vi "ShapeokoV3.vi"() -> ()   [LabVIEW 2024]
uses:
  <vilib>/Instr/_visa.llb/VISA Configure Serial Port (Instr).vi
  Subs/ShapekoGlobal.vi
panel:
  out "position":cluster{"X (inch)":dbl, "Y (inch)":dbl} {"X (inch)" format="%#.2g"; "Y (inch)" format="%#.2g"}
  out "position":cluster{"X (mm)":dbl, "Y (mm)":dbl}
  out "unlocked":bool
  in  "desired":cluster{"X":dbl, "Y":dbl, "Z":dbl}
  in  "Controls":T1
  in  "Jog":T2={"X-"=FALSE, "X+"=FALSE, "Y-"=FALSE, "Y+"=FALSE, "Z_"=FALSE, "Z+"=FALSE, "Dist"=1000, "Feed"=500} {"Feed" items=["100 mm/min"=100, "200 mm/min"=200, "300 mm/min"=300, "400 mm/min"=400, "500 mm/min"=500]; "Dist" items=["0.1 mm"=1, "1 mm"=10, "10 mm"=100, "100 mm"=1000]}
  in  "SubCut":cluster{dbl, dbl}(slide)={1.0, 0.0} scale=0.0..1.0
  out "(inch)":T3 {"Z Max" format="%#.3f"; "Z Min" format="%#.3f"; "Y Max" format="%#.3f"; "Y Min" format="%#.3f"; "X Max" format="%#.3f"; "X Min" format="%#.3f"}
  in  "Setup":T4={"Scaling (pixels/mm)"=1.0, "Tool Diameter (inch)"=0.25, "Origin location"={"x (mm)"=10, "y (mm)"=300}, "Wood dim"={"width (inch)"=10.0, "height (inch)"=12.0}}
  out "Tool Loc":picture
  in  "Path":path
  in  "Run":bool
  out "Cut":picture
  out "Bounds (mm)":T3 {"Z Max" format="%#.1f"; "Z Min" format="%#.1f"; "Y Max" format="%#.1f"; "Y Min" format="%#.1f"; "X Max" format="%#.1f"; "X Min" format="%#.1f"}
  out "Position":T5
  in  "stop":bool
  in  "VISA":refnum<visa-resource-name>="ASRL3::INSTR"
  in  "Cmds":i32(listbox)=-1
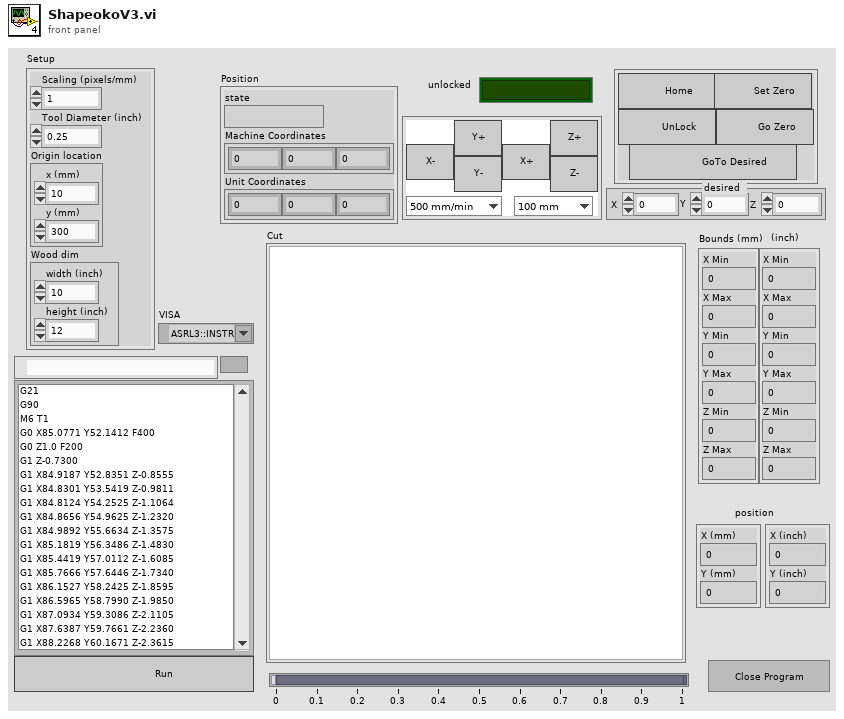
[diagram p1: front panel]
types:
  T1 = cluster{"Home Button":bool, "Set zero":bool, "Lock Button":bool, "Goto Zero":bool, "Goto Desired":bool}
  T2 = cluster{"X-":bool, "X+":bool, "Y-":bool, "Y+":bool, "Z_":bool, "Z+":bool, "Dist":u16, "Feed":u16}
  T3 = cluster{"X Min":dbl, "X Max":dbl, "Y Min":dbl, "Y Max":dbl, "Z Min":dbl, "Z Max":dbl}
  T4 = cluster{"Scaling (pixels/mm)":dbl, "Tool Diameter (inch)":dbl, "Origin location":cluster{"x (mm)":i16, "y (mm)":i16}, "Wood dim":cluster{"width (inch)":dbl, "height (inch)":dbl}}
  T5 = cluster{"state":string, "Machine Coordinates":cluster{"X":dbl, "Y":dbl, "Z":dbl}, "Unit Coordinates":cluster{"X":dbl, "Y":dbl, "Z":dbl}}
  T6 = typedef "LVPositionTypeDef.ctl" = cluster{"Left":i32, "Top":i32}
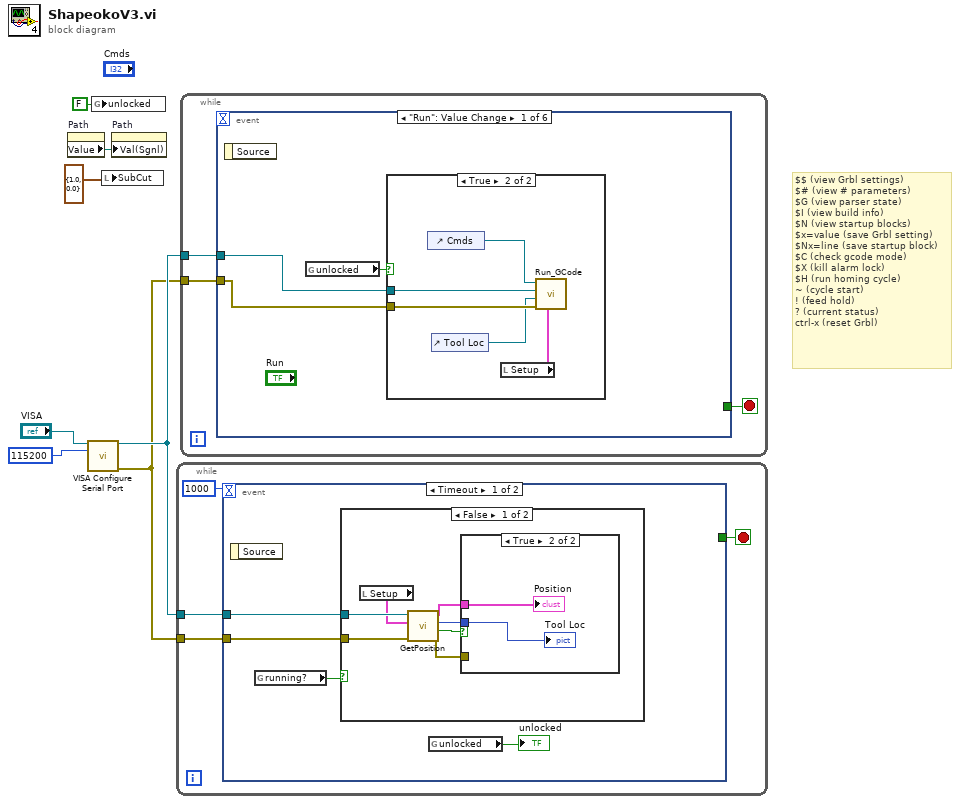
[diagram p0: block diagram]
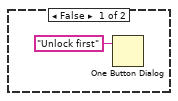
[diagram p2: hidden frame]
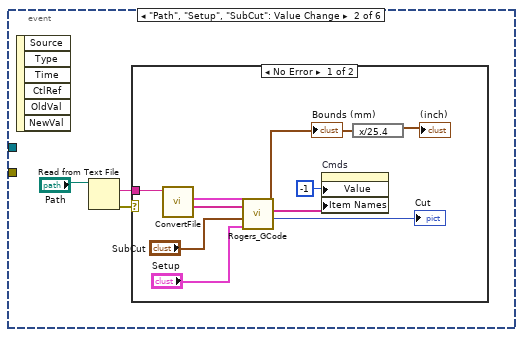
[diagram p3: hidden frame]
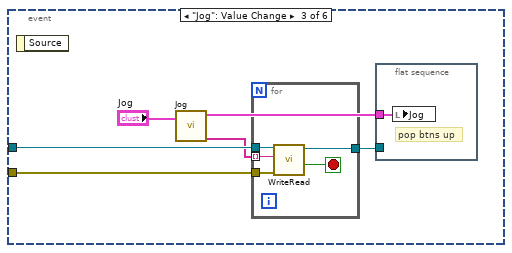
[diagram p5: hidden frame]
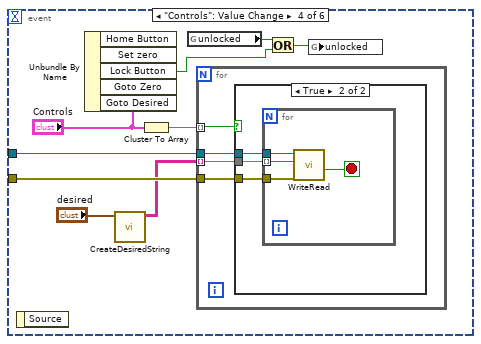
[diagram p6: hidden frame]
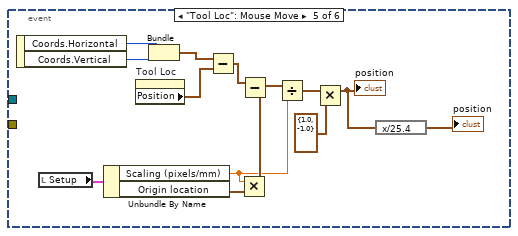
[diagram p8: hidden frame]
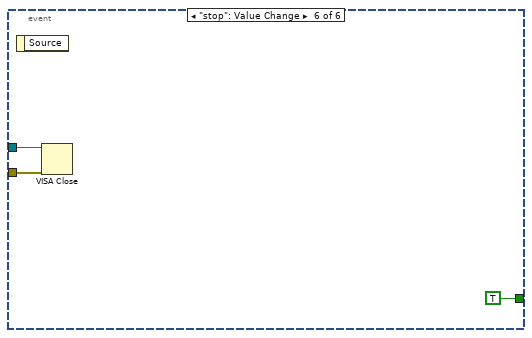
[diagram p9: hidden frame]
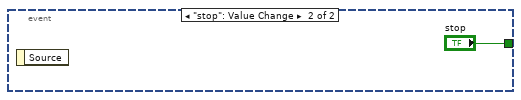
[diagram p12: hidden frame]
diagram:
  # "$$ (view Grbl settings)\n$# (view # parameters)\n$G (view parser state)\n$I (view build info)\n$N (view startup blocks)\n$x=value (save Grbl setting)\n$Nx=line (save startup block)\n$C (check gcode mode)\n$X (kill alarm lock)\n$H (run homing cycle)\n~ (cycle start)\n! (feed hold)\n? (current status)\nctrl-x (reset Grbl)"
  n1 = property on="Path" class="Path"() -> ("Value"=w2:path)  [unwired: 2 in, 2 out]
  n2 = call-poly "VISA Configure Serial Port"("VISA resource name"="VISA", "baud rate (9600)"=u32 115200 ("Baud")) -> ("VISA resource name out"=w5:refnum<visa-resource-name>, "error out"=w4:errorcluster)  [unwired: 12 in]
  n3 = global write "ShapekoGlobal.vi" "unlocked"(FALSE ("Locked")) -> ()
  n4 = local write "SubCut"(cluster{dbl, dbl} {1.0, 0.0} ("SubCut")) -> ()
  n5 = property on="Path" class="Path"("Val(Sgnl)"=w2) -> ()  [unwired: 2 in, 2 out]
  n6 = while {
    tunnel: w5 -> [w11]
    tunnel: w4 -> [w10]
    stop <- w8 stop-if-true
    n7 = event shown="[0] Timeout" {
      selector: _ -> [_ _]
      dyn-events: _ -> [_ _]
      timeout: u32 1000 ("milliseconds to wait") -> [_ _]
      tunnel: w11 -> [w15 _]
      tunnel: w10 -> [w14 _]
      tunnel: [_ "stop"] -> w8
      event Timeout {
        n8 = event-data() -> ()  [unwired: 1 in, 1 out]
        n9 = global read "ShapekoGlobal.vi" "running?"() -> (w12:bool)
        n10 = case shown="False" w12 {
          tunnel: w15 -> [w22 _]
          tunnel: w14 -> [w21 _]
          frame False {
            n11 = local read "Setup"() -> (w16:T4)
            n12 = call "GetPosition.vi"("error in (no error)"=w21, "Setup"=w16, "VISA Refnum in"=w22) -> ("error out"=w18:errorcluster, "success?"=w19:bool, "new picture"=w17:picture, "Position"=w20:T5)  [unwired: 5 in]
            n13 = case shown="True" w19 {
              tunnel: w20 -> [_ w24]
              tunnel: w18 -> [_ _]
              tunnel: w17 -> [_ w23]
              frame False {
              }
              frame True {
                "Position" <- w24
                "Tool Loc" <- w23
              }
            }
          }
          frame True {
          }
        }
        n14 = global read "ShapekoGlobal.vi" "unlocked"() -> (→"unlocked":bool)
      }
      event "stop": Value Change {
        n15 = event-data() -> ()  [unwired: 1 in, 1 out]
      }
    }
  }
  n16 = while {
    tunnel: w5 -> [w28]
    tunnel: w4 -> [w27]
    stop <- w26 stop-if-true
    n17 = event shown="[0] \"Run\": Value Change" {
      selector: _ -> [_ _ _ _ _ _]
      dyn-events: _ -> [_ _ _ _ _ _]
      timeout: _ -> [_ _ _ _ _ _]
      tunnel: w28 -> [w31 _ w56 w69 _ w98]
      tunnel: w27 -> [w30 _ w52 w68 _ w99]
      tunnel: [_ _ _ _ _ TRUE] -> w26
      event "Run": Value Change {
        n18 = event-data() -> ()  [unwired: 1 in, 1 out]
        n19 = global read "ShapekoGlobal.vi" "unlocked"() -> (w29:bool)
        n20 = case shown="True" w29 {
          tunnel: w31 -> [_ w37]
          tunnel: w30 -> [_ w36]
          frame False {
            n21 = One Button Dialog(message="Unlock first") -> ()  [unwired: 1 in, 1 out]
          }
          frame True {
            n22 = control-ref of="Cmds"() -> (w35:refnum<vi>)
            n23 = control-ref of="Tool Loc"() -> (w34:refnum<vi>)
            n24 = local read "Setup"() -> (w33:T4)
            n25 = call "Run_GCode.vi"("Setup"=w33, "error in (no error)"=w36, "Tool Refnum"=w34, "VISA resource name in"=w37, "ListBox in"=w35) -> ()  [unwired: 7 in]
          }
        }
      }
      event "Path", "Setup", "SubCut": Value Change {
        n26 = event-data() -> ()  [unwired: 1 in, 6 out]
        n27 = Read from Text File(file (use dialog)="Path") -> (text=w40:string, error out=w39:errorcluster)  [unwired: 3 in, 2 out]
        n28 = case shown="No Error" w39 {
          tunnel: w40 -> [w50 _]
          frame No Error {
            n29 = call "ConvertFile.vi"("String"=w50) -> ("Commands"=w47:string[], "cmd amd State"=w46:cluster{"Command":string, "End State":dbl[]}[])  [unwired: 8 in, 1 out]
            n30 = call "Rogers_GCode.vi"("cmd amd State"=w46, "Setup"="Setup", "SubCut"="SubCut", "Commands in"=w47) -> ("Cut"=→"Cut":picture, "Commands"=w49:string[], "Bounds"=w44:T3)  [unwired: 5 in]
            "Bounds (mm)" <- w44
            n31 = property on="Cmds" class="LstBox (strict)"("Value"=-1 ("Cmds"), "Item Names"=w49) -> ()  [unwired: 2 in, 2 out]
            n32 = expression code="x/25.4"(w44) -> (→"(inch)":T3)
          }
          frame Error {
          }
        }
      }
      event "Jog": Value Change {
        n33 = event-data() -> ()  [unwired: 1 in, 1 out]
        n34 = call "Jog.vi"("Jog"="Jog") -> ("Commands"=w55:string[], "output cluster"=w53:T2)  [unwired: 8 in, 1 out]
        n35 = for {
          tunnel: w55 -> [w62] mode=indexing
          tunnel: w56 -> [w61]
          tunnel: w52 -> [w60]
          tunnel: [w59] -> w51
          stop <- w58 stop-if-true
          n36 = call "WriteRead.vi"("error in (no error)"=w60, "String in"=w62, "VISA Refnum in"=w61) -> ("warned"=w58:bool, "VISA Refnum out"=w59:refnum<visa-resource-name>)  [unwired: 5 in, 2 out]
        }
        n37 = flat-sequence {
          tunnel: w53 -> [w57]
          tunnel: w51 -> [_]
          frame #0 {
            # "pop btns up"
            n38 = local write "Jog"(w57) -> ()
          }
        }
      }
      event "Controls": Value Change {
        n39 = event-data() -> ()  [unwired: 1 in, 1 out]
        n40 = Unbundle By Name("Controls") -> ("Lock Button"=w64:bool)  [unwired: 4 out]
        n41 = call "CreateDesiredString.vi"("desired"="desired") -> ("cmds"=w67:string[][])  [unwired: 10 in]
        n42 = Cluster To Array(cluster="Controls") -> (array=w71:bool[])
        n43 = global read "ShapekoGlobal.vi" "unlocked"() -> (w65:bool)
        n44 = for {
          tunnel: w71 -> [w75] mode=indexing
          tunnel: w69 -> [w74]
          tunnel: w68 -> [w73]
          tunnel: w67 -> [w72] mode=indexing
          n45 = case shown="True" w75 {
            tunnel: w74 -> [_ w78]
            tunnel: w73 -> [_ w77]
            tunnel: w72 -> [_ w76]
            frame False {
            }
            frame True {
              n46 = for {
                tunnel: w78 -> [w82]
                tunnel: w77 -> [w81]
                tunnel: w76 -> [w80] mode=indexing
                stop <- w79 stop-if-true
                n47 = call "WriteRead.vi"("error in (no error)"=w81, "String in"=w80, "VISA Refnum in"=w82) -> ("warned"=w79:bool)  [unwired: 5 in, 3 out]
              }
            }
          }
        }
        n48 = Or(x=w65, y=w64) -> (x .or. y?=w63:bool)
        n49 = global write "ShapekoGlobal.vi" "unlocked"(w63) -> ()
      }
      event "Tool Loc": Mouse Move {
        n50 = event-data() -> ("Coords.Horizontal"=w96:i32, "Coords.Vertical"=w95:i32)  [unwired: 1 in]
        n51 = local read "Setup"() -> (w92:T4)
        n52 = Unbundle By Name(w92) -> ("Scaling (pixels/mm)"=w89:dbl, "Origin location"=w93:cluster{"x (mm)":i16, "y (mm)":i16})
        n53 = property on="Tool Loc" class="Pict"() -> ("Position"=w87:T6)  [unwired: 2 in, 2 out]
        n54 = Bundle("Horizontal"=w96, "Vertical"=w95) -> (w88:cluster{"Horizontal":i32, "Vertical":i32})  [unwired: 1 in]
        n55 = Subtract(x=w88, y=w87) -> (x-y=w86:T6)
        n56 = Multiply(x=w89, y=w93) -> (x*y=w91:cluster{"x (mm)":dbl, "y (mm)":dbl})
        n57 = Subtract(x=w86, y=w91) -> (x-y=w90:cluster{dbl, dbl})
        n58 = Divide(x=w90, y=w89) -> (x/y=w94:cluster{dbl, dbl})
        n59 = Multiply(x=w94, y=cluster{dbl, dbl} {1.0, -1.0}) -> (x*y=w84:cluster{dbl, dbl})
        "position" <- w84
        n60 = expression code="x/25.4"(w84) -> (→"position":cluster{dbl, dbl})
      }
      event "stop": Value Change {
        n61 = event-data() -> ()  [unwired: 1 in, 1 out]
        n62 = VISA Close(VISA resource name=w98, error in (no error)=w99) -> ()  [unwired: 1 out]
      }
    }
  }
